vi "picoharp_replace_file_extension.vi"(10 "new_extension":string=".stream", 11 "input_file":path) -> (3 "new_name":path)   [LabVIEW 2015, in "picoharp.lvclass"]
uses:
  picoharp.lvclass
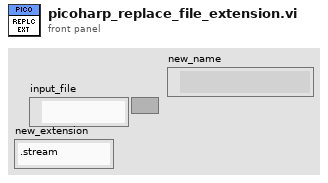
[diagram p1: front panel]
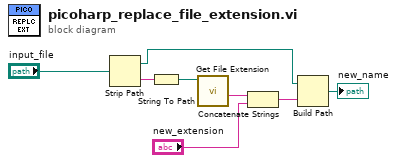
[diagram p0: block diagram]
diagram:
  n1 = Strip Path(path="input_file") -> (stripped path=w3:path, name=w6:string)
  n2 = String To Path(string=w6) -> (path=w5:path)
  n3 = call <vilib>:"Get File Extension.vi"("file"=w5) -> ("filename without extension"=w7:string)  [unwired: 6 in, 4 out]
  n4 = Concatenate Strings(w7, "new_extension") -> (w8:string)
  n5 = Build Path(base path=w3, name or relative path=w8) -> (appended path=→"new_name":path)
